vi "Template RF Test Fetch Results.vi"(8 "error in (no error)":errorcluster, 11 "Template Tx Test in":refnum<class "Template RF Test.lvclass">) -> (0 "error out":errorcluster, 2 "Default USL":T1, 3 "Template Tx Test out":refnum<class "Template RF Test.lvclass">)   [LabVIEW 2015, in "niDTS Template.lvlib" / "Template RF Test.lvclass"]
uses:
  Template RF Test.lvclass
  Includes/Template RF Test INC Results.ctl
  niDTS Template.lvlib
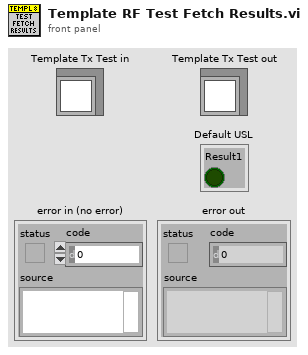
[diagram p1: front panel]
types:
  T1 = typedef "niDTS Template.lvlib/Template RF Test INC Results.ctl" = cluster{"Result1":bool}
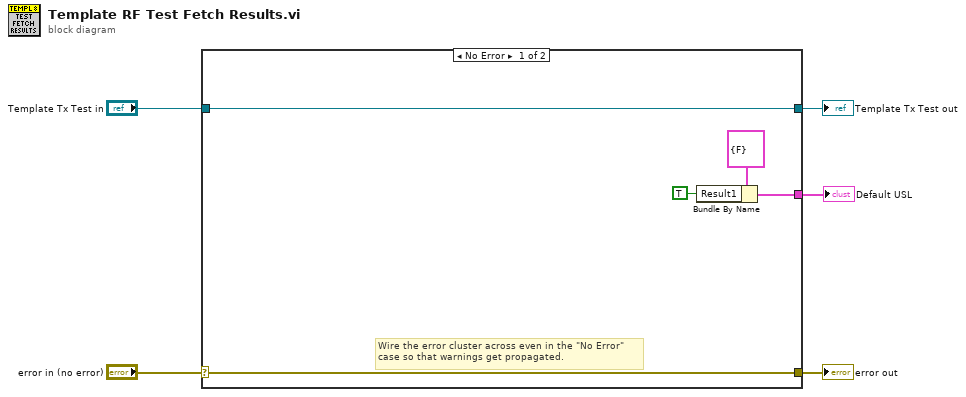
[diagram p0: block diagram]
diagram:
  n1 = case shown="No Error" "error in (no error)" {
    selector: "error in (no error)" -> [w10 w12]
    tunnel: [w10 w12] -> w4
    tunnel: [w9 w11] -> w2
    tunnel: "Template Tx Test in" -> [w9 w11]
    tunnel: [w7 _] -> w1
    frame No Error {
      # "Wire the error cluster across even in the \"No Error\"\ncase so that warnings get propagated."
      n2 = Bundle By Name(cluster=T1 {"Result1"=FALSE} ("Default LSL"), "Result1"=TRUE) -> (w7:T1)
    }
    frame Error {
    }
  }
  "error out" <- w4
  "Template Tx Test out" <- w2
  "Default USL" <- w1
